vi "TangoSelectPos.vi"(7 "TANGO ID":i32, 8 "error in (no error)":errorcluster, 9 "Button":string, 10 "ItemNames":string[][](array[string]), 11 "Enum in":refnum<vi>) -> (0 "error out":errorcluster, 3 "Queue out":refnum<queue>)   [LabVIEW 2018]
uses:
  <userlib>/Tango_DLL/Tango_DLL.lvlib
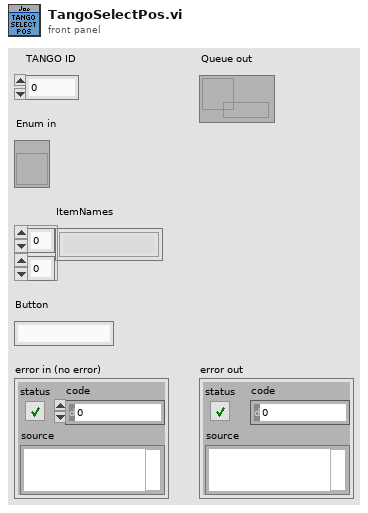
[diagram p1: front panel]
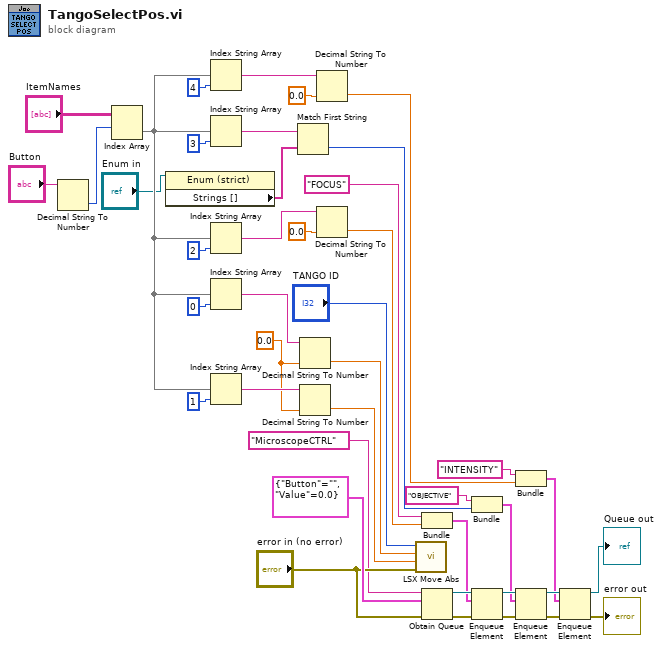
[diagram p0: block diagram]
diagram:
  w11 = 0.0
  n1 = Decimal String To Number(string="Button") -> (number=w4:i32)  [unwired: 2 in, 1 out]
  n2 = Index Array(array="ItemNames", index (row)=w4) -> (element=w42:string[])  [unwired: 1 in]
  n3 = property on="Property Node" class="Enum (strict)"(reference="Enum in") -> ("Strings []"=w26:string[])  [unwired: 1 in, 2 out]
  n4 = Index String Array(1:4 ("index"), 2:w42) -> (0:w33:string)  [unwired: 1 in]
  n5 = Index String Array(1:3 ("index"), 2:w42) -> (0:w27:string)  [unwired: 1 in]
  n6 = Index String Array(1:2 ("index"), 2:w42) -> (0:w16:string)  [unwired: 1 in]
  n7 = Index String Array(1:0 ("index"), 2:w42) -> (0:w10:string)  [unwired: 1 in]
  n8 = Index String Array(1:1 ("index"), 2:w42) -> (0:w14:string)  [unwired: 1 in]
  n9 = Match First String(2:w26, 3:w27) -> (0:w32:i32)  [unwired: 1 out]
  n10 = Decimal String To Number(string=w10, default (0L)=w11) -> (number=w13:dbl)  [unwired: 1 in, 1 out]
  n11 = Decimal String To Number(string=w14, default (0L)=w11) -> (number=w15:dbl)  [unwired: 1 in, 1 out]
  n12 = Decimal String To Number(string=w33, default (0L)=0.0 ("default (0 I32)")) -> (number=w35:dbl)  [unwired: 1 in, 1 out]
  n13 = Decimal String To Number(string=w16, default (0L)=0.0 ("default (0 I32)")) -> (number=w20:dbl)  [unwired: 1 in, 1 out]
  n14 = call <userlib>:"LSX Move Abs.vi"("error in (no error)"="error in (no error)", "dY"=w15, "dX"=w13, "lLSID"="TANGO ID") -> ()  [unwired: 6 in, 2 out]
  n15 = Bundle("FOCUS", w20) -> (w21:cluster{string, dbl})  [unwired: 1 in]
  n16 = Obtain Queue(name (unnamed)="MicroscopeCTRL", element data type=cluster{"Button":string, "Value":dbl} {"Button"="", "Value"=0.0}, error in (no error)="error in (no error)") -> (queue out=w22:refnum<queue>, error out=w23:errorcluster)  [unwired: 2 in, 1 out]
  n17 = Bundle("OBJECTIVE", "index"=w32) -> (w29:cluster{string, "index":i32})  [unwired: 1 in]
  n18 = Enqueue Element(queue=w22, element=w21, error in (no error)=w23) -> (queue out=w31:refnum<queue>, error out=w30:errorcluster)  [unwired: 1 in, 1 out]
  n19 = Bundle("INTENSITY", w35) -> (w37:cluster{string, dbl})  [unwired: 1 in]
  n20 = Enqueue Element(queue=w31, element=w29, error in (no error)=w30) -> (queue out=w40:refnum<queue>, error out=w41:errorcluster)  [unwired: 1 in, 1 out]
  n21 = Enqueue Element(queue=w40, element=w37, error in (no error)=w41) -> (queue out=→"Queue out":refnum<queue>, error out=→"error out":errorcluster)  [unwired: 1 in, 1 out]
